vi "PH_Tektronix_7000.Save Data 2 Harddisk.vi"(0 "i ref in":refnum<vi>, 5 "error in":errorcluster) -> (14 "i ref out":refnum<vi>, 19 "error out":errorcluster)   [LabVIEW 2014, in "PH_Tektronix_7000.lvlib"]
doc: "This VI saves the data stored at own attributes to the harddisk."
uses:
  PH_Tektronix_7000.lvlib
  PH_Basics/PH_Common/Names/PH_Names.File Types.ctl
  PH_Basics/PH_Common/PH_Common.lvlib
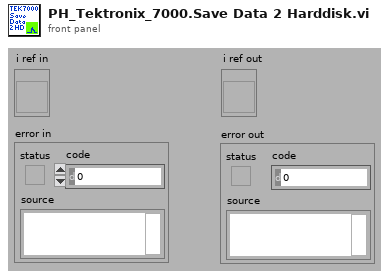
[diagram p1: front panel]
types:
  T1 = typedef "PH_Common.lvlib/PH_Names.File Types.ctl" = string
  T2 = typedef "PH_Tektronix_7000.lvlib/PH_Tektronix_7000.i attribute.ctl" = cluster{"VISA Resource Name":refnum<visa-resource-name>, "IDN":cluster{"Instrument Driver":string, "Instrument Firmware":string, "Model":string, "Serial Number":string}, "Selftest":cluster{"Result":i32, "Message":string}, "Trigger Configuration":T3, "Acquisition Configuration":T4, "GUI Refs":T5, "State":T6, "Error Message":string, "Allow Prdc Loop?":bool, "Channel 1":T7, "Channel 2":T7, "Channel 3":T7, "Channel 4":T7, "Data CH 1":waveform(dbl), "Data CH 2":waveform(dbl), "Data CH 3":waveform(dbl), "Data CH 4":waveform(dbl), "Allow config?":bool, "Name Channel 1":string, "Name Channel 2":string, "Name Channel 3":string, "Name Channel 4":string, "Fetch Data before sending to PSDB?":bool, "Constructor passed?":bool, "Data taken at":timestamp, "Plot Colors":u32[], "Default VISA Resource":string}
  T3 = typedef "PH_Tektronix_7000.lvlib/PH_Tektronix_7000.Trigger Config.ctl" = cluster{"Source":u16, "Level [V]":dbl, "Slope":u16, "Coupling":u16, "Trigger Mode":u16}
  T4 = typedef "PH_Tektronix_7000.lvlib/PH_Tektronix_7000.Acquisition Config.ctl" = cluster{"Record Length":u32, "Timebase [s/div]":dbl, "Position [%]":dbl, "Acquisition Type":u16, "Average Waveforms":i32, "Envelope Waveforms":i32, "WfmDB Samples":i32, "Continuous?":bool, "Delay [s]":dbl, "Run?":bool}
  T5 = typedef "PH_Tektronix_7000.lvlib/PH_Tektronix_7000.GUI Refs.ctl" = cluster{"Graph":refnum<vi>, "State":refnum<vi>, "Delete":refnum<vi>, "VISA Resource":refnum<vi>, "Allow Configure":refnum<vi>, "Fetch Data":refnum<vi>, "Fetch before sending Data to PSDB":refnum<vi>, "Name Channel 1":refnum<vi>, "Name Channel 2":refnum<vi>, "Name Channel 3":refnum<vi>, "Name Channel 4":refnum<vi>, "Prdc Intervall [ms]":refnum<vi>, "Data taken":refnum<vi>, "Model":refnum<vi>, "Serial Number":refnum<vi>, "Firmware":refnum<vi>, "Driver":refnum<vi>, "Acquisition":refnum<vi>, "Trigger":refnum<vi>, "Cursor: D Time [s]":refnum<vi>, "Cursor: D Signal [V]":refnum<vi>, "Channel 1":refnum<vi>, "Channel 2":refnum<vi>, "Channel 3":refnum<vi>, "Channel 4":refnum<vi>}
  T6 = typedef "PH_StatusHandler.lvlib/PH_StatusHandler.Status.ctl" = i16
  T7 = typedef "PH_Tektronix_7000.lvlib/PH_Tektronix_7000.Channel Config.ctl" = cluster{"Enable Channel":bool, "Bandwidth":u16, "Input Impedance":u16, "Vertical Coupling":u16, "Probe Attenuation":dbl, "Range [V/div]":dbl, "Position [div]":dbl, "Bandwidth raw":string}
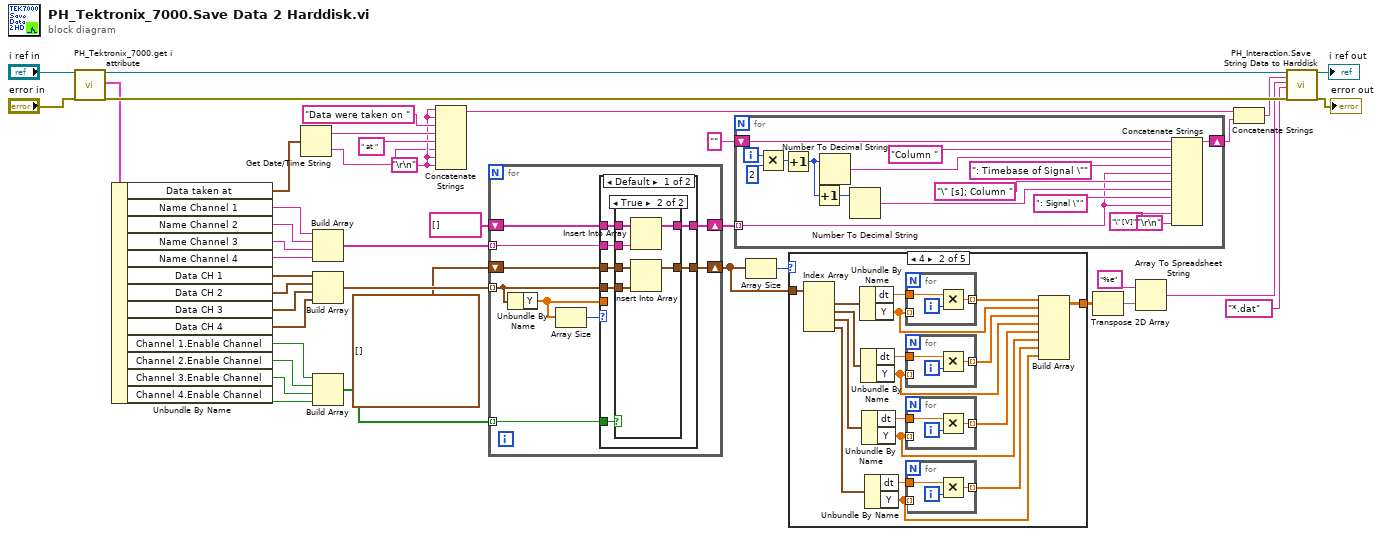
[diagram p0: block diagram]
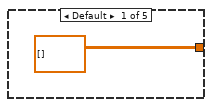
[diagram p2: hidden frame]
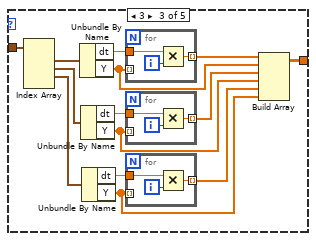
[diagram p3: hidden frame]
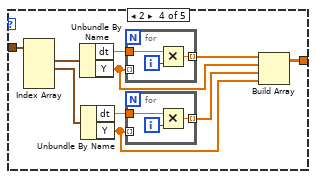
[diagram p4: hidden frame]
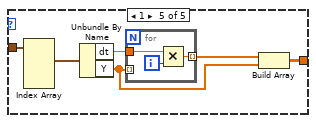
[diagram p5: hidden frame]
diagram:
  w7 = "\r\n"
  n1 = call "PH_Tektronix_7000.get i attribute.vi"("i ref in"="i ref in", "error in (no error)"="error in") -> ("i ref out"=w14:refnum<vi>, "i attribute"=w16:T2, "error out"=w38:errorcluster)  [unwired: 15 in]
  n2 = Unbundle By Name(w16) -> ("Data taken at"=w11:timestamp, "Name Channel 1"=w20:string, "Name Channel 2"=w21:string, "Name Channel 3"=w22:string, "Name Channel 4"=w24:string, "Data CH 1"=w36:waveform(dbl), "Data CH 2"=w35:waveform(dbl), "Data CH 3"=w34:waveform(dbl), "Data CH 4"=w33:waveform(dbl), "Channel 1.Enable Channel"=w29:bool, "Channel 2.Enable Channel"=w26:bool, "Channel 3.Enable Channel"=w27:bool, "Channel 4.Enable Channel"=w28:bool)
  n3 = Get Date/Time String(seconds (now)=w11) -> (date string=w9:string, time string=w5:string)  [unwired: 2 in]
  n4 = Build Array(w20, w21, w22, w24) -> (w23:string[])
  n5 = Build Array(w36, w35, w34, w33) -> (w32:waveform(dbl)[])
  n6 = Build Array(w29, w26, w27, w28) -> (w25:bool[])
  n7 = Concatenate Strings(w7, w7, "Data were taken on " ("string"), w9, " at " ("string"), w5, w7, w7) -> (w6:string)
  n8 = for {
    tunnel: w25 -> [w43] mode=indexing
    tunnel: w32 -> [w44] mode=indexing
    tunnel: w23 -> [w50] mode=indexing
    shift-right: [w49] -> w3
    shift-left: string[] [] -> [w48]
    shift-right: [w46] -> w19
    shift-left: waveform(dbl)[] [] -> [w45]
    n9 = Unbundle By Name(w44) -> ("Y"=w47:dbl[])
    n10 = Array Size(array=w47) -> (size(s)=w51:i32)
    n11 = case shown="Default" w51 {
      tunnel: w50 -> [w58 _]
      tunnel: [w57 w68] -> w49
      tunnel: w48 -> [w56 w68]
      tunnel: w47 -> [_ _]
      tunnel: [w55 w67] -> w46
      tunnel: w45 -> [w54 w67]
      tunnel: w44 -> [w53 _]
      tunnel: w43 -> [w52 _]
      frame Default {
        n12 = case shown="True" w52 {
          tunnel: w58 -> [_ w66]
          tunnel: [w60 w65] -> w57
          tunnel: w56 -> [w60 w64]
          tunnel: [w59 w63] -> w55
          tunnel: w54 -> [w59 w62]
          tunnel: w53 -> [_ w61]
          frame False {
          }
          frame True {
            n13 = Insert Into Array(array=w64, new element=w66) -> (w65:string[])  [unwired: 1 in]
            n14 = Insert Into Array(array=w62, new element=w61) -> (w63:waveform(dbl)[])  [unwired: 1 in]
          }
        }
      }
      frame 0 {
      }
    }
  }
  n15 = for {
    tunnel: w3 -> [w75] mode=indexing
    shift-right: [w84] -> w1
    shift-left: "" -> [w83]
    i -> [w71]
    n16 = Multiply(x=w71, y=2) -> (x*y=w70:i32)
    n17 = Increment(x=w70) -> (x+1=w69:i32)
    n18 = Increment(x=w69) -> (x+1=w81:i32)
    n19 = Number To Decimal String(number=w69) -> (decimal integer string=w80:string)  [unwired: 1 in]
    n20 = Number To Decimal String(number=w81) -> (decimal integer string=w77:string)  [unwired: 1 in]
    n21 = Concatenate Strings(w83, "Column " ("string"), w80, ": Timebase of Signal \"" ("string"), w75, "\" [s]; Column " ("string"), w77, ": Signal \"" ("string"), w75, "\" [V]" ("string"), "\r\n") -> (w84:string)
  }
  n22 = Array Size(array=w19) -> (size(s)=w18:i32)
  n23 = case shown="4" w18 {
    tunnel: w19 -> [_ w103 w129 w148 w160]
    tunnel: [dbl[][] [] w95 w122 w142 w155] -> w17
    frame Default {
    }
    frame 4 {
      n24 = Index Array(array=w103) -> (element #1=w101:waveform(dbl), element #2=w98:waveform(dbl), element #3=w97:waveform(dbl), element #4=w96:waveform(dbl))  [unwired: 4 in]
      n25 = Unbundle By Name(w101) -> ("dt"=w102:dbl, "Y"=w99:dbl[])
      n26 = Unbundle By Name(w98) -> ("dt"=w94:dbl, "Y"=w93:dbl[])
      n27 = Unbundle By Name(w97) -> ("dt"=w92:dbl, "Y"=w91:dbl[])
      n28 = Unbundle By Name(w96) -> ("dt"=w90:dbl, "Y"=w86:dbl[])
      n29 = for {
        tunnel: w102 -> [w114]
        tunnel: [w115] -> w100 mode=indexing
        tunnel: w99 -> [_] mode=indexing
        i -> [w113]
        n30 = Multiply(x=w114, y=w113) -> (x*y=w115:dbl)
      }
      n31 = for {
        tunnel: w94 -> [w111]
        tunnel: [w112] -> w89 mode=indexing
        tunnel: w93 -> [_] mode=indexing
        i -> [w110]
        n32 = Multiply(x=w111, y=w110) -> (x*y=w112:dbl)
      }
      n33 = for {
        tunnel: w92 -> [w108]
        tunnel: [w109] -> w88 mode=indexing
        tunnel: w91 -> [_] mode=indexing
        i -> [w107]
        n34 = Multiply(x=w108, y=w107) -> (x*y=w109:dbl)
      }
      n35 = for {
        tunnel: w90 -> [w105]
        tunnel: [w106] -> w87 mode=indexing
        tunnel: w86 -> [_] mode=indexing
        i -> [w104]
        n36 = Multiply(x=w105, y=w104) -> (x*y=w106:dbl)
      }
      n37 = Build Array(w100, w99, w89, w93, w88, w91, w87, w86) -> (w95:dbl[][])
    }
    frame 3 {
      n38 = Index Array(array=w129) -> (element #1=w127:waveform(dbl), element #2=w124:waveform(dbl), element #3=w123:waveform(dbl))  [unwired: 4 in, 1 out]
      n39 = Unbundle By Name(w127) -> ("dt"=w128:dbl, "Y"=w125:dbl[])
      n40 = Unbundle By Name(w124) -> ("dt"=w121:dbl, "Y"=w120:dbl[])
      n41 = Unbundle By Name(w123) -> ("dt"=w119:dbl, "Y"=w118:dbl[])
      n42 = for {
        tunnel: w128 -> [w137]
        tunnel: [w138] -> w126 mode=indexing
        tunnel: w125 -> [_] mode=indexing
        i -> [w136]
        n43 = Multiply(x=w137, y=w136) -> (x*y=w138:dbl)
      }
      n44 = for {
        tunnel: w121 -> [w134]
        tunnel: [w135] -> w117 mode=indexing
        tunnel: w120 -> [_] mode=indexing
        i -> [w133]
        n45 = Multiply(x=w134, y=w133) -> (x*y=w135:dbl)
      }
      n46 = for {
        tunnel: w119 -> [w131]
        tunnel: [w132] -> w116 mode=indexing
        tunnel: w118 -> [_] mode=indexing
        i -> [w130]
        n47 = Multiply(x=w131, y=w130) -> (x*y=w132:dbl)
      }
      n48 = Build Array(w126, w125, w117, w120, w116, w118) -> (w122:dbl[][])
    }
    frame 2 {
      n49 = Index Array(array=w148) -> (element #1=w146:waveform(dbl), element #2=w143:waveform(dbl))  [unwired: 4 in, 2 out]
      n50 = Unbundle By Name(w146) -> ("dt"=w147:dbl, "Y"=w144:dbl[])
      n51 = Unbundle By Name(w143) -> ("dt"=w141:dbl, "Y"=w140:dbl[])
      n52 = for {
        tunnel: w147 -> [w153]
        tunnel: [w154] -> w145 mode=indexing
        tunnel: w144 -> [_] mode=indexing
        i -> [w152]
        n53 = Multiply(x=w153, y=w152) -> (x*y=w154:dbl)
      }
      n54 = for {
        tunnel: w141 -> [w150]
        tunnel: [w151] -> w139 mode=indexing
        tunnel: w140 -> [_] mode=indexing
        i -> [w149]
        n55 = Multiply(x=w150, y=w149) -> (x*y=w151:dbl)
      }
      n56 = Build Array(w145, w144, w139, w140) -> (w142:dbl[][])
    }
    frame 1 {
      n57 = Index Array(array=w160) -> (element #1=w158:waveform(dbl))  [unwired: 4 in, 3 out]
      n58 = Unbundle By Name(w158) -> ("dt"=w159:dbl, "Y"=w156:dbl[])
      n59 = for {
        tunnel: w159 -> [w162]
        tunnel: [w163] -> w157 mode=indexing
        tunnel: w156 -> [_] mode=indexing
        i -> [w161]
        n60 = Multiply(x=w162, y=w161) -> (x*y=w163:dbl)
      }
      n61 = Build Array(w157, w156) -> (w155:dbl[][])
    }
  }
  n62 = Transpose 2D Array(2D array=w17) -> (transposed array=w41:dbl[][])
  n63 = Array To Spreadsheet String(array=w41, 3:"%e" ("format string")) -> (spreadsheet string=w15:string)  [unwired: 1 in]
  n64 = Concatenate Strings(w6, w1) -> (w4:string)
  n65 = call "PH_Interaction.Save String Data to Harddisk.vi"("i ref in"=w14, "Explanation (for Example: Column 1: xxx, ...)"=w4, "Data (for example: Columns)"=w15, "file name extension"=T1 "*.dat" ("file name extinction"), "error in (no error)"=w38) -> ("i ref out"=→"i ref out":refnum<vi>, "error out"=→"error out":errorcluster)  [unwired: 12 in, 1 out]
